vi "HEWH Set Draw Stations.vi"(7 "Draw States":T1, 8 "Error In":errorcluster, 11 "Station":string) -> (0 "Error Out":errorcluster, 3 "result string":string)   [LabVIEW 2019]
uses:
  Type Definitions/HEWH Set Draw States.ctl
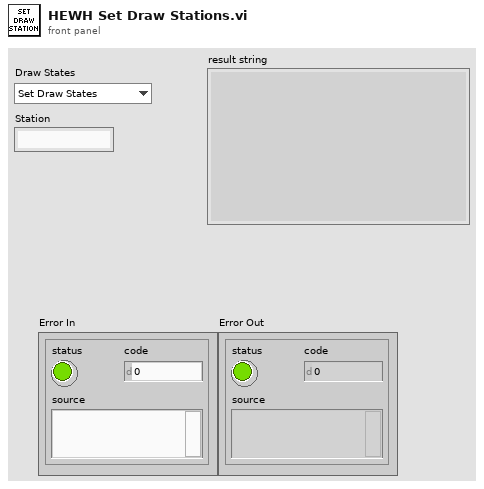
[diagram p1: front panel]
types:
  T1 = typedef "HEWH Set Draw States.ctl" = enum16{"Set Draw States", "Temperature Decline"}
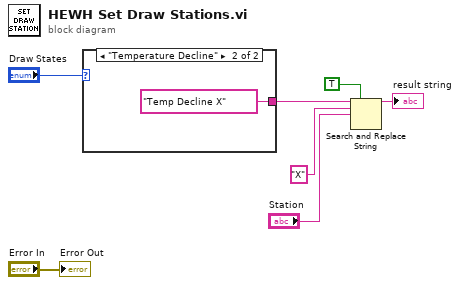
[diagram p0: block diagram]
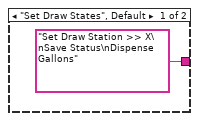
[diagram p2: hidden frame]
diagram:
  n1 = case shown="\"Temperature Decline\"" "Draw States" {
    tunnel: ["Set Draw Station >> X\nSave Status\nDispense Gallons" "Temp Decline X"] -> w5
    frame "Set Draw States", Default {
    }
    frame "Temperature Decline" {
    }
  }
  n2 = Search and Replace String(replace all?=TRUE ("replace all? (F)"), input string=w5, search string="X", replace string="Station") -> (result string=→"result string":string)  [unwired: 4 in, 3 out]
  "Error Out" <- "Error In"
